vi "Return Items.vi"(10 "Selection":enum16{"Selection", "All"}(ring), 11 "REFERENCES":T1) -> ()   [LabVIEW 2019]
uses:
  Controls/References Cluster.ctl
  Controls/Custom Calendar/Custom Calendar.xctl
  Controls/Table Data Types/Inventory Data Type.ctl
  Controls/Table Data Types/Checked In Archive Data Type.ctl
  Controls/Column Names/Inventory Column Names.ctl
  <vilib>/addons/database/Connection.llb/DB Tools Open Connec (String).vi
  <vilib>/addons/database/_DB Variant To Data/Database Variant To Data.xnode
  <vilib>/addons/database/NI_Database_API.lvlib
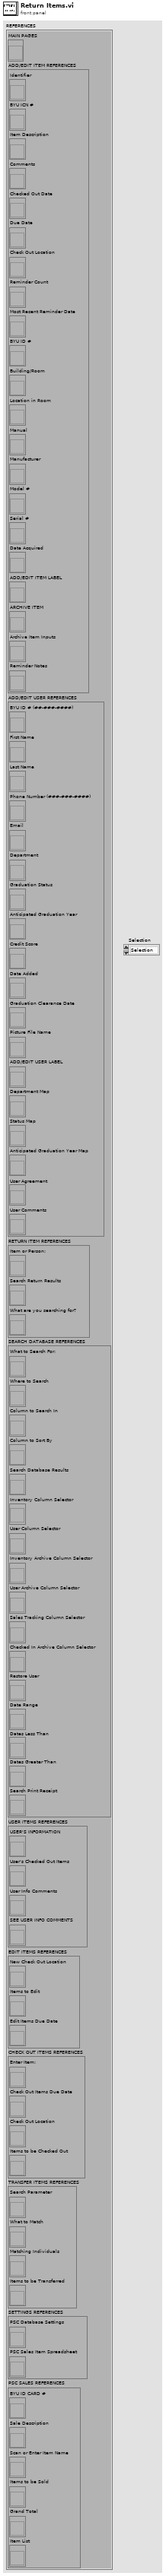
[diagram p1: front panel]
types:
  T1 = typedef "References Cluster.ctl" = cluster{"MAIN PAGES":refnum<vi>, "ADD/EDIT ITEM REFERENCES":cluster{"Identifier":refnum<vi>, "BYU ICN #":refnum<vi>, "Item Description":refnum<vi>, "Comments":refnum<vi>, "Checked Out Date":refnum<vi>, "Due Date":refnum<vi>, "Check Out Location":refnum<vi>, "Reminder Count":refnum<vi>, "Most Recent Reminder Date":refnum<vi>, "BYU ID #":refnum<vi>, "Building/Room":refnum<vi>, "Location in Room":refnum<vi>, "Manual":refnum<vi>, "Manufacturer":refnum<vi>, "Model #":refnum<vi>, "Serial #":refnum<vi>, "Date Acquired":refnum<vi>, "ADD/EDIT ITEM LABEL":refnum<vi>, "ARCHIVE ITEM":refnum<vi>, "Archive Item Inputs":refnum<vi>, "Reminder Notes":refnum<vi>}, "ADD/EDIT USER REFERENCES":cluster{"BYU ID # (##-###-####)":refnum<vi>, "First Name":refnum<vi>, "Last Name":refnum<vi>, "Phone Number (###-###-####)":refnum<vi>, "Email":refnum<vi>, "Department":refnum<vi>, "Graduation Status":refnum<vi>, "Anticipated Graduation Year":refnum<vi>, "Credit Score":refnum<vi>, "Date Added":refnum<vi>, "Graduation Clearance Date":refnum<vi>, "Picture File Name":refnum<vi>, "ADD/EDIT USER LABEL":refnum<vi>, "Department Map":refnum<vi>, "Status Map":refnum<vi>, "Anticipated Graduation Year Map":refnum<vi>, "User Agreement":refnum<vi>, "User Comments":refnum<vi>}, "RETURN ITEM REFERENCES":cluster{"Item or Person:":refnum<vi>, "Search Return Results":refnum<vi>, "What are you searching for?":refnum<vi>}, "SEARCH DATABASE REFERENCES":cluster{"What to Search For:":refnum<vi>, "Where to Search":refnum<vi>, "Column to Search In":refnum<vi>, "Column to Sort By":refnum<vi>, "Search Database Results":refnum<vi>, "Inventory Column Selector":refnum<vi>, "User Column Selector":refnum<vi>, "Inventory Archive Column Selector":refnum<vi>, "User Archive Column Selector":refnum<vi>, "Sales Tracking Column Selector":refnum<vi>, "Checked In Archive Column Selector":refnum<vi>, "Restore User":refnum<vi>, "Date Range":refnum<vi>, "Dates Less Than":refnum<vi>, "Dates Greater Than":refnum<vi>, "Search Print Receipt":refnum<vi>}, "USER ITEMS REFERENCES":cluster{"USER'S INFORMATION":refnum<vi>, "User's Checked Out Items":refnum<vi>, "User Info Comments":refnum<vi>, "SEE USER INFO COMMENTS":refnum<vi>}, "EDIT ITEMS REFERENCES":cluster{"New Check Out Location":refnum<vi>, "Items to Edit":refnum<vi>, "Edit Items Due Date":refnum<vi>}, "CHECK OUT ITEMS REFERENCES":cluster{"Enter Item:":refnum<vi>, "Check Out Items Due Date":refnum<vi>, "Check Out Location":refnum<vi>, "Items to be Checked Out":refnum<vi>}, "TRANSFER ITEMS REFERENCES":cluster{"Search Parameter":refnum<vi>, "What to Match":refnum<vi>, "Matching Individuals":refnum<vi>, "Items to be Transferred":refnum<vi>}, "SETTINGS REFERENCES":cluster{"PSC Database Settings":refnum<vi>, "PSC Sales Item Spreadsheet":refnum<vi>}, "PSC SALES REFERENCES":cluster{"BYU ID CARD #":refnum<vi>, "Sale Description":refnum<vi>, "Scan or Enter Item Name":refnum<vi>, "Items to be Sold":refnum<vi>, "Grand Total":refnum<vi>, "Item List":refnum<vi>}}
  T2 = cluster{"USER'S INFORMATION":refnum<vi>, "User's Checked Out Items":refnum<vi>, "User Info Comments":refnum<vi>, "SEE USER INFO COMMENTS":refnum<vi>}
  T3 = typedef "NI_Database_API.lvlib/Conn ObjectReference.ctl" = refnum<k1>
  T4 = typedef "Inventory Data Type.ctl" = cluster{"Identifier":string, "BYU ICN #":string, "Item Description":string, "Comments":string, "Checked Out Date":string, "Due Date":string, "Check Out Location":string, "Reminder Count":i32, "Most Recent Reminder Date":string, "BYU ID #":string, "Building/Room":string, "Location in Room":string, "Manual":string, "Manufacturer":string, "Model #":string, "Serial #":string, "Date Acquired":string, "Reminder Notes":string}
  T5 = typedef "Checked In Archive Data Type.ctl" = cluster{"Identifier":string, "BYU ICN #":string, "Item Description":string, "Comments":string, "Checked Out Date":string, "Due Date":string, "Check Out Location":string, "Reminder Count":i32, "Most Recent Reminder Date":string, "BYU ID #":string, "Building/Room":string, "Location in Room":string, "Manual":string, "Manufacturer":string, "Model #":string, "Serial #":string, "Date Acquired":string, "Date Returned":string, "Reminder Notes":string}
  T6 = typedef "Inventory Column Names.ctl" = string[]
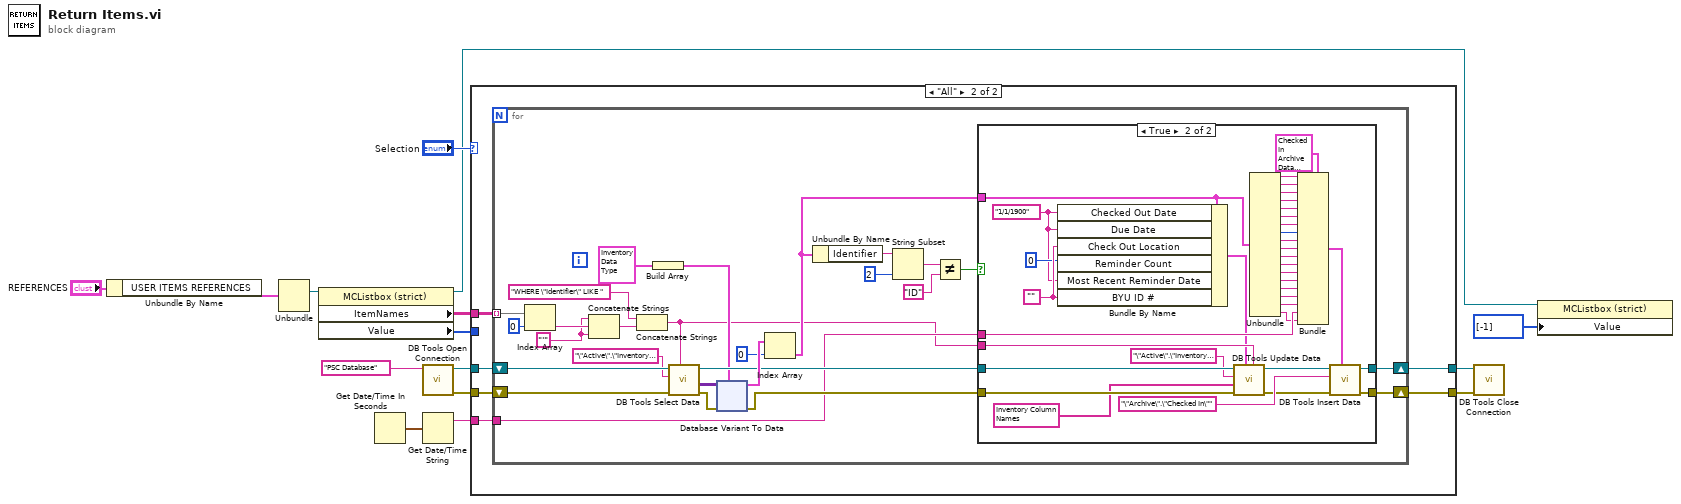
[diagram p0: block diagram]
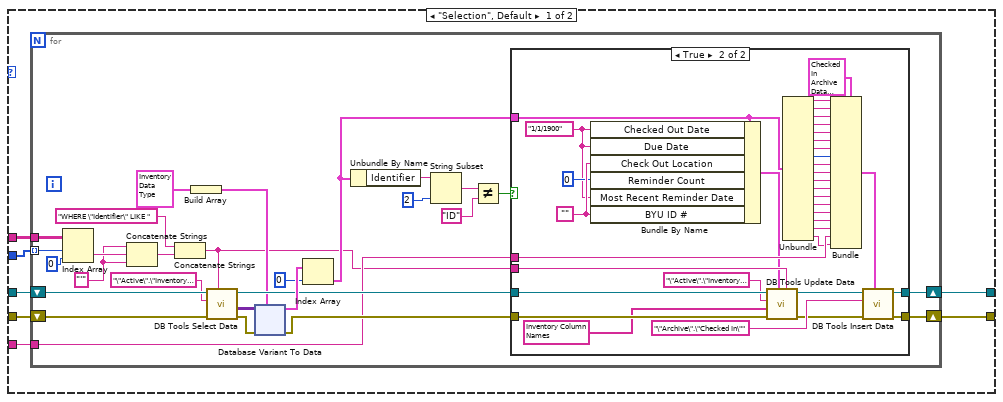
[diagram p2: hidden frame]
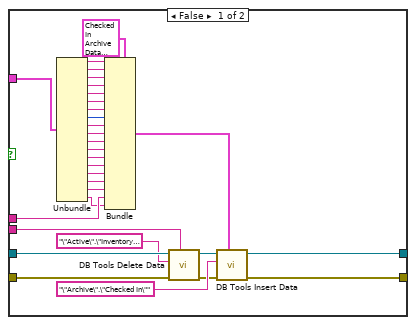
[diagram p3: hidden frame]
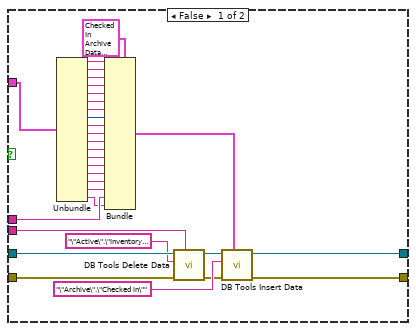
[diagram p4: hidden frame]
diagram:
  n1 = Unbundle By Name("REFERENCES") -> ("USER ITEMS REFERENCES"=w3:T2)
  n2 = Unbundle(w3) -> ("User's Checked Out Items"=w13:refnum<vi>)  [unwired: 3 out]
  n3 = property class="MCListbox (strict)"(reference=w13) -> (reference out=w2:refnum<vi>, "ItemNames"=w12:string[][], "Value"=w11:i32[])  [unwired: 1 in, 1 out]
  n4 = Get Date/Time In Seconds() -> (seconds since 1Jan1904=w7:timestamp)
  n5 = call-poly <vilib>:"DB Tools Open Connection.vi"("connection information"="PSC Database") -> ("error out"=w9:errorcluster, "connection reference"=w10:T3)  [unwired: 7 in]
  n6 = Get Date/Time String(seconds (now)=w7) -> (date string=w8:string)  [unwired: 2 in, 1 out]
  n7 = case shown="\"All\"" "Selection" {
    tunnel: w12 -> [w20 w690]
    tunnel: w11 -> [w19 _]
    tunnel: w10 -> [w22 w687]
    tunnel: w9 -> [w21 w686]
    tunnel: w8 -> [w18 w691]
    tunnel: [w17 w689] -> w6
    tunnel: [w16 w688] -> w5
    frame "Selection", Default {
      n8 = for {
        tunnel: w19 -> [w49] mode=indexing
        tunnel: w20 -> [w50]
        shift-right: [w35] -> w17
        shift-left: w22 -> [w48]
        shift-right: [w34] -> w16
        shift-left: w21 -> [w47]
        tunnel: w18 -> [w36]
        w28 = "'"
        n9 = Index Array(array=w50, index (row)=w49, index (col)=0 ("disabled index (col)")) -> (element=w29:string)
        n10 = Concatenate Strings(w28, w29, w28) -> (w30:string)
        n11 = Concatenate Strings("WHERE \"Identifier\" LIKE " ("string"), w30) -> (w23:string)
        n12 = Build Array(T4 {"Identifier"="", "BYU ICN #"="", "Item Description"="", "Comments"="", "Checked Out Date"="", "Due Date"="", "Check Out Location"="", "Reminder Count"=0, "Most Recent Reminder Date"="", "BYU ID #"="", "Building/Room"="", "Location in Room"="", "Manual"="", "Manufacturer"="", "Model #"="", "Serial #"="", "Date Acquired"="", "Reminder Notes"=""} ("Array")) -> (w32:T4[])
        n13 = call <vilib>:"DB Tools Select Data.vi"("condition"=w23, "error in (no error)"=w47, "table"="\"Active\".\"Inventory\"", "connection reference"=w48) -> ("error out"=w43:errorcluster, "data"=w44:variant[][], "connection reference out"=w37:T3)  [unwired: 2 in]
        n14 = xnode "Database Variant To Data"("database variant"=w44, "error in (no error)"=w43, "type"=w32) -> ("data"=w42:T4[], "error out"=w38:errorcluster)
        n15 = Index Array(array=w42, index=0) -> (element=w39:T4)
        n16 = Unbundle By Name(w39) -> ("Identifier"=w26:string)
        n17 = String Subset(string=w26, length (rest)=2 ("length (rest)")) -> (substring=w27:string)  [unwired: 1 in]
        n18 = Not Equal?(x=w27, y="ID" ("regular expression")) -> (x != y?=w40:bool)
        n19 = case shown="True" w40 {
          tunnel: w39 -> [w74 w85]
          tunnel: w38 -> [w79 w97]
          tunnel: w37 -> [w81 w99]
          tunnel: w23 -> [w78 w96]
          tunnel: w36 -> [w56 w100]
          tunnel: [w54 w88] -> w35
          tunnel: [w53 w87] -> w34
          frame False {
            n20 = Unbundle(w74) -> ("Identifier"=w73:string, "BYU ICN #"=w72:string, "Item Description"=w71:string, "Comments"=w70:string, "Checked Out Date"=w69:string, "Due Date"=w68:string, "Check Out Location"=w67:string, "Reminder Count"=w66:i32, "Most Recent Reminder Date"=w65:string, "BYU ID #"=w64:string, "Building/Room"=w63:string, "Location in Room"=w62:string, "Manual"=w61:string, "Manufacturer"=w60:string, "Model #"=w59:string, "Serial #"=w58:string, "Date Acquired"=w57:string, "Reminder Notes"=w51:string)
            n21 = Bundle(cluster=T5 {"Identifier"="", "BYU ICN #"="", "Item Description"="", "Comments"="", "Checked Out Date"="", "Due Date"="", "Check Out Location"="", "Reminder Count"=0, "Most Recent Reminder Date"="", "BYU ID #"="", "Building/Room"="", "Location in Room"="", "Manual"="", "Manufacturer"="", "Model #"="", "Serial #"="", "Date Acquired"="", "Date Returned"="", "Reminder Notes"=""} ("CHECKED IN ARCHIVE DATA TYPE"), "Identifier"=w73, "BYU ICN #"=w72, "Item Description"=w71, "Comments"=w70, "Checked Out Date"=w69, "Due Date"=w68, "Check Out Location"=w67, "Reminder Count"=w66, "Most Recent Reminder Date"=w65, "BYU ID #"=w64, "Building/Room"=w63, "Location in Room"=w62, "Manual"=w61, "Manufacturer"=w60, "Model #"=w59, "Serial #"=w58, "Date Acquired"=w57, "Date Returned"=w56, "Reminder Notes"=w51) -> (w55:T5)
            n22 = call <vilib>:"DB Tools Delete Data.vi"("condition"=w78, "error in (no error)"=w79, "table"="\"Active\".\"Inventory\"", "connection reference"=w81) -> ("error out"=w75:errorcluster, "connection reference out"=w76:T3)  [unwired: 6 in]
            n23 = call <vilib>:"DB Tools Insert Data.vi"("data"=w55, "error in (no error)"=w75, "table"="\"Archive\".\"Checked In\"", "connection reference"=w76) -> ("error out"=w53:errorcluster, "connection reference out"=w54:T3)  [unwired: 6 in]
          }
          frame True {
            w84 = "1/1/1900" ("Checked Out Date")
            w95 = ""
            n24 = Bundle By Name(cluster=w85, "Checked Out Date"=w84, "Due Date"=w84, "Check Out Location"=w95, "Reminder Count"=0 ("# of Reminders Sent"), "Most Recent Reminder Date"=w84, "BYU ID #"=w95) -> (w93:T4)
            n25 = call <vilib>:"DB Tools Update Data.vi"("condition"=w96, "data"=w93, "error in (no error)"=w97, "columns"=T6 ["\"Identifier\"", "\"BYU ICN #\"", "\"Item Description\"", "\"Comments\"", "\"Checked Out Date\"", "\"Due Date\"", "\"Check Out Location\"", "\"Reminder Count\"", "\"Most Recent Reminder Date\"", "\"BYU ID #\"", "\"Building/Room\"", "\"Location in Room\"", "\"Manual\"", "\"Manufacturer\"", "\"Model #\"", "\"Serial #\"", "\"Date Acquired\"", "\"Reminder Notes\""] ("INVENTORY COLUMN NAMES"), "table"="\"Active\".\"Inventory\"", "connection reference"=w99) -> ("error out"=w89:errorcluster, "connection reference out"=w90:T3)  [unwired: 4 in]
            n26 = Unbundle(w85) -> ("Identifier"=w117:string, "BYU ICN #"=w116:string, "Item Description"=w115:string, "Comments"=w114:string, "Checked Out Date"=w113:string, "Due Date"=w112:string, "Check Out Location"=w111:string, "Reminder Count"=w110:i32, "Most Recent Reminder Date"=w109:string, "BYU ID #"=w108:string, "Building/Room"=w107:string, "Location in Room"=w106:string, "Manual"=w105:string, "Manufacturer"=w104:string, "Model #"=w103:string, "Serial #"=w102:string, "Date Acquired"=w101:string, "Reminder Notes"=w83:string)
            n27 = Bundle(cluster=T5 {"Identifier"="", "BYU ICN #"="", "Item Description"="", "Comments"="", "Checked Out Date"="", "Due Date"="", "Check Out Location"="", "Reminder Count"=0, "Most Recent Reminder Date"="", "BYU ID #"="", "Building/Room"="", "Location in Room"="", "Manual"="", "Manufacturer"="", "Model #"="", "Serial #"="", "Date Acquired"="", "Date Returned"="", "Reminder Notes"=""} ("CHECKED IN ARCHIVE DATA TYPE"), "Identifier"=w117, "BYU ICN #"=w116, "Item Description"=w115, "Comments"=w114, "Checked Out Date"=w113, "Due Date"=w112, "Check Out Location"=w111, "Reminder Count"=w110, "Most Recent Reminder Date"=w109, "BYU ID #"=w108, "Building/Room"=w107, "Location in Room"=w106, "Manual"=w105, "Manufacturer"=w104, "Model #"=w103, "Serial #"=w102, "Date Acquired"=w101, "Date Returned"=w100, "Reminder Notes"=w83) -> (w92:T5)
            n28 = call <vilib>:"DB Tools Insert Data.vi"("data"=w92, "error in (no error)"=w89, "table"="\"Archive\".\"Checked In\"", "connection reference"=w90) -> ("error out"=w87:errorcluster, "connection reference out"=w88:T3)  [unwired: 6 in]
          }
        }
      }
    }
    frame "All" {
      n29 = for {
        tunnel: w690 -> [w718] mode=indexing
        shift-right: [w706] -> w689
        shift-left: w687 -> [w717]
        shift-right: [w705] -> w688
        shift-left: w686 -> [w716]
        tunnel: w691 -> [w703]
        w698 = "'"
        n30 = Index Array(array=w718, index=0 ("disabled index (col)")) -> (element=w699:string)
        n31 = Concatenate Strings(w698, w699, w698) -> (w700:string)
        n32 = Concatenate Strings("WHERE \"Identifier\" LIKE " ("string"), w700) -> (w692:string)
        n33 = Build Array(T4 {"Identifier"="", "BYU ICN #"="", "Item Description"="", "Comments"="", "Checked Out Date"="", "Due Date"="", "Check Out Location"="", "Reminder Count"=0, "Most Recent Reminder Date"="", "BYU ID #"="", "Building/Room"="", "Location in Room"="", "Manual"="", "Manufacturer"="", "Model #"="", "Serial #"="", "Date Acquired"="", "Reminder Notes"=""} ("Array")) -> (w701:T4[])
        n34 = call <vilib>:"DB Tools Select Data.vi"("condition"=w692, "error in (no error)"=w716, "table"="\"Active\".\"Inventory\"", "connection reference"=w717) -> ("error out"=w712:errorcluster, "data"=w713:variant[][], "connection reference out"=w707:T3)  [unwired: 2 in]
        n35 = xnode "Database Variant To Data"("database variant"=w713, "error in (no error)"=w712, "type"=w701) -> ("data"=w711:T4[], "error out"=w708:errorcluster)
        n36 = Index Array(array=w711, index=0) -> (element=w694:T4)
        n37 = Unbundle By Name(w694) -> ("Identifier"=w697:string)
        n38 = String Subset(string=w697, length (rest)=2 ("length (rest)")) -> (substring=w696:string)  [unwired: 1 in]
        n39 = Not Equal?(x=w696, y="ID" ("regular expression")) -> (x != y?=w709:bool)
        n40 = case shown="True" w709 {
          tunnel: w694 -> [w720 w762]
          tunnel: w708 -> [w747 w765]
          tunnel: w707 -> [w749 w767]
          tunnel: w692 -> [w746 w764]
          tunnel: w703 -> [w725 w768]
          tunnel: [w723 w756] -> w706
          tunnel: [w722 w755] -> w705
          frame False {
            n41 = Unbundle(w720) -> ("Identifier"=w742:string, "BYU ICN #"=w741:string, "Item Description"=w740:string, "Comments"=w739:string, "Checked Out Date"=w738:string, "Due Date"=w737:string, "Check Out Location"=w736:string, "Reminder Count"=w735:i32, "Most Recent Reminder Date"=w734:string, "BYU ID #"=w733:string, "Building/Room"=w732:string, "Location in Room"=w731:string, "Manual"=w730:string, "Manufacturer"=w729:string, "Model #"=w728:string, "Serial #"=w727:string, "Date Acquired"=w726:string, "Reminder Notes"=w719:string)
            n42 = Bundle(cluster=T5 {"Identifier"="", "BYU ICN #"="", "Item Description"="", "Comments"="", "Checked Out Date"="", "Due Date"="", "Check Out Location"="", "Reminder Count"=0, "Most Recent Reminder Date"="", "BYU ID #"="", "Building/Room"="", "Location in Room"="", "Manual"="", "Manufacturer"="", "Model #"="", "Serial #"="", "Date Acquired"="", "Date Returned"="", "Reminder Notes"=""} ("CHECKED IN ARCHIVE DATA TYPE"), "Identifier"=w742, "BYU ICN #"=w741, "Item Description"=w740, "Comments"=w739, "Checked Out Date"=w738, "Due Date"=w737, "Check Out Location"=w736, "Reminder Count"=w735, "Most Recent Reminder Date"=w734, "BYU ID #"=w733, "Building/Room"=w732, "Location in Room"=w731, "Manual"=w730, "Manufacturer"=w729, "Model #"=w728, "Serial #"=w727, "Date Acquired"=w726, "Date Returned"=w725, "Reminder Notes"=w719) -> (w724:T5)
            n43 = call <vilib>:"DB Tools Delete Data.vi"("condition"=w746, "error in (no error)"=w747, "table"="\"Active\".\"Inventory\"", "connection reference"=w749) -> ("error out"=w743:errorcluster, "connection reference out"=w744:T3)  [unwired: 6 in]
            n44 = call <vilib>:"DB Tools Insert Data.vi"("data"=w724, "error in (no error)"=w743, "table"="\"Archive\".\"Checked In\"", "connection reference"=w744) -> ("error out"=w722:errorcluster, "connection reference out"=w723:T3)  [unwired: 6 in]
          }
          frame True {
            w752 = "1/1/1900" ("Checked Out Date")
            w763 = ""
            n45 = Bundle By Name(cluster=w762, "Checked Out Date"=w752, "Due Date"=w752, "Check Out Location"=w763, "Reminder Count"=0, "Most Recent Reminder Date"=w752, "BYU ID #"=w763) -> (w761:T4)
            n46 = call <vilib>:"DB Tools Update Data.vi"("condition"=w764, "data"=w761, "error in (no error)"=w765, "columns"=T6 ["\"Identifier\"", "\"BYU ICN #\"", "\"Item Description\"", "\"Comments\"", "\"Checked Out Date\"", "\"Due Date\"", "\"Check Out Location\"", "\"Reminder Count\"", "\"Most Recent Reminder Date\"", "\"BYU ID #\"", "\"Building/Room\"", "\"Location in Room\"", "\"Manual\"", "\"Manufacturer\"", "\"Model #\"", "\"Serial #\"", "\"Date Acquired\"", "\"Reminder Notes\""] ("INVENTORY COLUMN NAMES"), "table"="\"Active\".\"Inventory\"", "connection reference"=w767) -> ("error out"=w757:errorcluster, "connection reference out"=w758:T3)  [unwired: 4 in]
            n47 = Unbundle(w762) -> ("Identifier"=w785:string, "BYU ICN #"=w784:string, "Item Description"=w783:string, "Comments"=w782:string, "Checked Out Date"=w781:string, "Due Date"=w780:string, "Check Out Location"=w779:string, "Reminder Count"=w778:i32, "Most Recent Reminder Date"=w777:string, "BYU ID #"=w776:string, "Building/Room"=w775:string, "Location in Room"=w774:string, "Manual"=w773:string, "Manufacturer"=w772:string, "Model #"=w771:string, "Serial #"=w770:string, "Date Acquired"=w769:string, "Reminder Notes"=w751:string)
            n48 = Bundle(cluster=T5 {"Identifier"="", "BYU ICN #"="", "Item Description"="", "Comments"="", "Checked Out Date"="", "Due Date"="", "Check Out Location"="", "Reminder Count"=0, "Most Recent Reminder Date"="", "BYU ID #"="", "Building/Room"="", "Location in Room"="", "Manual"="", "Manufacturer"="", "Model #"="", "Serial #"="", "Date Acquired"="", "Date Returned"="", "Reminder Notes"=""} ("CHECKED IN ARCHIVE DATA TYPE"), "Identifier"=w785, "BYU ICN #"=w784, "Item Description"=w783, "Comments"=w782, "Checked Out Date"=w781, "Due Date"=w780, "Check Out Location"=w779, "Reminder Count"=w778, "Most Recent Reminder Date"=w777, "BYU ID #"=w776, "Building/Room"=w775, "Location in Room"=w774, "Manual"=w773, "Manufacturer"=w772, "Model #"=w771, "Serial #"=w770, "Date Acquired"=w769, "Date Returned"=w768, "Reminder Notes"=w751) -> (w760:T5)
            n49 = call <vilib>:"DB Tools Insert Data.vi"("data"=w760, "error in (no error)"=w757, "table"="\"Archive\".\"Checked In\"", "connection reference"=w758) -> ("error out"=w755:errorcluster, "connection reference out"=w756:T3)  [unwired: 6 in]
          }
        }
      }
    }
  }
  n50 = call <vilib>:"DB Tools Close Connection.vi"("error in (no error)"=w5, "connection reference"=w6) -> ()  [unwired: 5 in, 1 out]
  n51 = property class="MCListbox (strict)"(reference=w2, "Value"=i32[] [-1]) -> ()  [unwired: 1 in, 2 out]
